vi "Standard INI Write Read.vi"(8 "error in":errorcluster, 11 "Editor Position in":refnum<class "Editor Position.lvclass">) -> (0 "error out":errorcluster, 3 "Editor Position out":refnum<class "Editor Position.lvclass">)   [LabVIEW 2020, in "Editor Position.lvclass"]
doc: "Tests a standard writing of the position to the INI file and reading it back."
uses:
  Editor Position.lvclass
  Editor Position.lvclass/Editor Position.ctl
  c60327dd-cdad-4b8c-8243-7f44ee2244ce.vi
  vi.lib/LabVIEW Icon API/lv_icon/lv_icon.lvlib
  <vilib>/Utility/miscctls.llb/LVRectTypeDef.ctl
  <vilib>/Astemes/LUnit/Test Case.lvclass
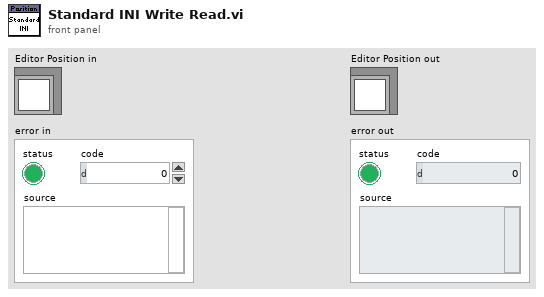
[diagram p1: front panel]
types:
  T1 = typedef "LVRectTypeDef.ctl" = cluster{"Left":i16, "Top":i16, "Right":i16, "Bottom":i16}
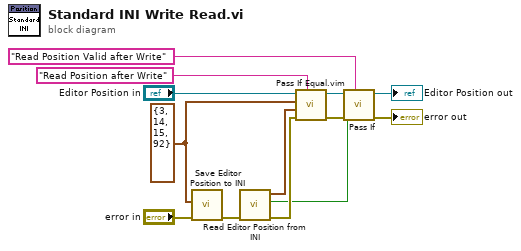
[diagram p0: block diagram]
diagram:
  w4 = T1 {"Left"=3, "Top"=14, "Right"=15, "Bottom"=92} ("Window Bounds")
  n1 = call "Save Editor Position to INI.vi"("error in"="error in", "Window Bounds"=w4) -> ("error out"=w11:errorcluster)  [unwired: 9 in]
  n2 = call "Read Editor Position from INI.vi"("error in"=w11) -> ("error out"=w12:errorcluster, "Bounds Valid"=w2:bool, "Window Bounds"=w3:T1)  [unwired: 7 in, 1 out]
  n3 = call "Pass If Equal.vim"("Description"="Read Position after Write", "error in (no error)"=w12, "Actual"=w3, "Expected"=w4, "LUnit Test Case In"="Editor Position in") -> ("error out"=w13:errorcluster, "LUnit Test Case Out"=w8:refnum<class "Editor Position.lvclass">)  [unwired: 5 in]
  n4 = call <vilib>:"Pass If.vi"("Description"="Read Position Valid after Write", "error in (no error)"=w13, "Pass?"=w2, "LUnit Test Case In"=w8) -> ("error out"=→"error out":errorcluster, "LUnit Test Case Out"=→"Editor Position out":refnum<class "Editor Position.lvclass">)  [unwired: 6 in]
